vi "Queue Self.vi"(9 "Priority?":bool, 10 "Msg Strategy":refnum<class "Msg Strategy.lvclass">, 11 "Base Event jettl in":refnum<class "Base Event jettl.lvclass">) -> (3 "Base Event jettl out":refnum<class "Base Event jettl.lvclass">)   [LabVIEW 2021, in "jettl.lvlib" / "Base Event jettl.lvlib" / "Base Event jettl.lvclass"]
uses:
  Base Event jettl.lvclass
  C:/git/jettl/src/jettl/jettl/jettl.lvclass
  Msg Strategy/Msg Strategy.lvclass
  Base Event jettl.lvclass/Base Event jettl.ctl
  jettl.lvlib
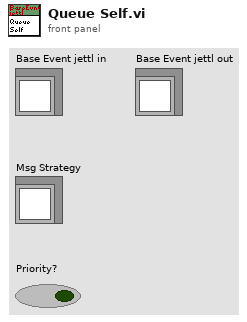
[diagram p1: front panel]
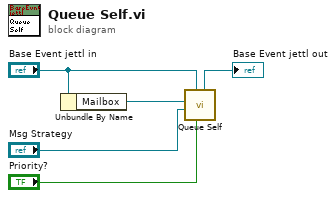
[diagram p0: block diagram]
diagram:
  n1 = Unbundle By Name("Base Event jettl in") -> ("Mailbox"=w5:refnum<data-value>)
  n2 = call "Queue Self.vi"("Priority?"="Priority?", "jettl in"="Base Event jettl in", "Msg Strategy"="Msg Strategy", "Queue Mailbox"=w5) -> ("jettl out"=→"Base Event jettl out":refnum<class "Base Event jettl.lvclass">)  [unwired: 7 in]
